vi "Handle Last Ack Core.vi"(4 "error in (no error)":errorcluster, 6 "Last Ack":refnum<class "Last Ack.lvclass">, 7 "SAS_AFTester_Template in":refnum<class "User Interface Tester.lvclass">) -> (0 "error out":errorcluster, 3 "SAS_AFTester_Template out":refnum<class "User Interface Tester.lvclass">)   [LabVIEW 2020, in "User Interface Tester.lvlib" / "User Interface Tester.lvclass"]
doc: "(<B>Filename</B>: Actor Framework.lvlib:Actor.lvclass:Handle Last Ack Core.vi)\n\nDefines how the caller actor responds to the Last Ack message from a nested actor. The Last Ack message is the final message a nested actor sends to its caller before it shuts down. The message contains information about the final state of the nested actor.\n\nBy default, this method does nothing except return any error the nested actor sent. A descendant class may override this method to define behavior."
uses:
  User Interface Tester.lvclass
  <vilib>/ActorFramework/LastAck/Last Ack.lvclass
  User Interface Tester.lvclass/User Interface Tester.ctl
  <vilib>/ActorFramework/Actor/Actor.lvclass
  <vilib>/SAS/Actor Tester/Enqueuer Manager/SAS_AFTester_Enqueuer Manager.lvclass
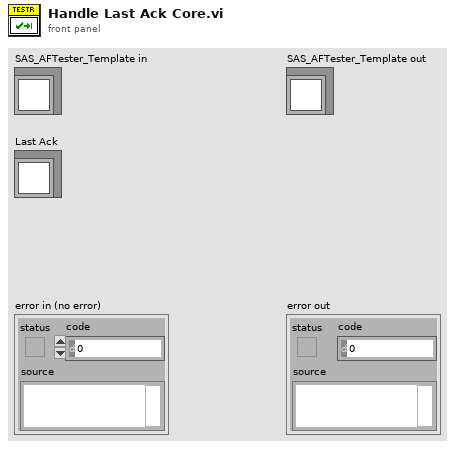
[diagram p1: front panel]
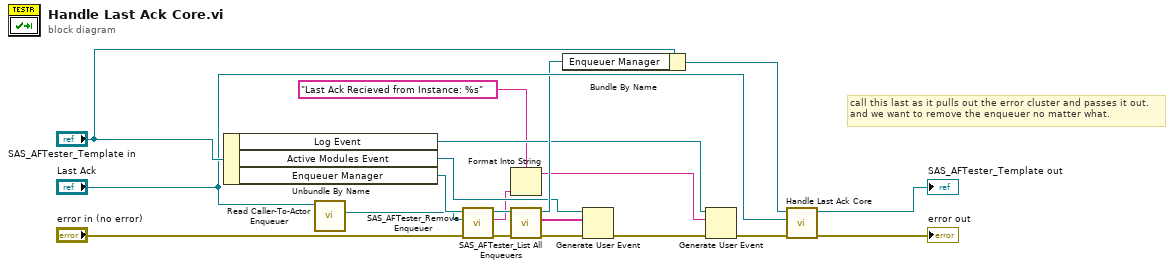
[diagram p0: block diagram]
diagram:
  # "call this last as it pulls out the error cluster and passes it out.\nand we want to remove the enqueuer no matter what."
  n1 = Unbundle By Name("SAS_AFTester_Template in") -> ("Log Event"=w6:refnum<user-event>, "Active Modules Event"=w8:refnum<user-event>, "Enqueuer Manager"=w17:refnum<class "SAS_AFTester_Enqueuer Manager.lvclass">)
  n2 = call <vilib>:"Read Caller-To-Actor Enqueuer.vi"("Last Ack"="Last Ack") -> ("Caller-to-Actor Enqueuer"=w13:refnum<class "Message Enqueuer.lvclass">)  [unwired: 10 in]
  n3 = call <vilib>:"SAS_AFTester_Remove Enqueuer.vi"("error in (no error)"="error in (no error)", "Message Enqueuer"=w13, "Enqueuer Manager in"=w17) -> ("error out"=w12:errorcluster, "ID of Deleted Element"=w2:string, "Enqueuer Manager out"=w11:refnum<class "SAS_AFTester_Enqueuer Manager.lvclass">)  [unwired: 6 in]
  n4 = Format Into String(format string="Last Ack Recieved from Instance: %s", w2) -> (resulting string=w1:string)  [unwired: 2 in, 1 out]
  n5 = call <vilib>:"SAS_AFTester_List All Enqueuers.vi"("error in (no error)"=w12, "Enqueuer Manager in"=w11) -> ("error out"=w9:errorcluster, "All Enqueuers"=w7:string[], "Enqueuer Manager out"=w10:refnum<class "SAS_AFTester_Enqueuer Manager.lvclass">)  [unwired: 7 in]
  n6 = Bundle By Name(cluster="SAS_AFTester_Template in", "Enqueuer Manager"=w10) -> (w15:refnum<class "User Interface Tester.lvclass">)
  n7 = Generate User Event(user event=w8, event data cluster=w7, error in=w9) -> (error out=w5:errorcluster)  [unwired: 1 in, 1 out]
  n8 = Generate User Event(user event=w6, event data cluster=w1, error in=w5) -> (error out=w4:errorcluster)  [unwired: 1 in, 1 out]
  n9 = call-parent "Handle Last Ack Core.vi"("error in (no error)"=w4, "Last Ack"="Last Ack", "Actor in"=w15) -> ("error out"=→"error out":errorcluster, "Actor out"=→"SAS_AFTester_Template out":refnum<class "User Interface Tester.lvclass">)  [unwired: 3 in]
